vi "Topo & GridSpectr_DriftCorrection_v10.vi"(6 "Internal use":string, 7 "Grid param":T1 {"height (m)" format="%#_6p"; "width (m)" format="%#_6p"; "center Y (m)" format="%#_6p"; "center X (m)" format="%#_6p"}, 8 "Error in (no error)":errorcluster, 9 "Points Y/Index Y":i32, 10 "Points X/Index X":i32, 11 "Method":enum16{"init", "run", "end"}(ring)=enum."end") -> (0 "Error out":errorcluster)   [LabVIEW 2014]
doc: "Example of a measurement VI to be used in the \"Experiments on a Grid\" tool as external VI.\n\nThis example measure the topography and spectroscopy data. The spectroscopy measurements are taken on a subgrid. The data are saved to a sxm and a binary file.\n\n- Nanonis Programming Interface -"
uses:
  <userlib>/Nanonis Prog Interface V5/Scan/Grid/GridPatternGet.vi
  <userlib>/Nanonis Prog Interface V5/Nanonis Prog Interface.lvlib
panel:
  in  "Lockin ON/OFF":bool
  in  "Correct Drift":bool
  in  "Email when finished":string="cornelius.krull@monash.edu"
  in  "STS z offset":dbl=1.15e-09 format="%#_6p"
  out "ETA":timestamp
  out "remaining":dbl format="%<%H:%M:%S>t"
  out "Progress":u8(slide) scale=0.0..100.0 scale format="%#.1g"
  out "total Points":i32
  in  "preSTS delay [ms]":u32=3
  in  "STS Bias":dbl=0.005 format="%#_6p"
  in  "Move Bias":dbl=-0.01 format="%#_6p"
  in  "Move Current":dbl=1.5e-11 format="%#_6p"
  in  "Imaging Bias":dbl=-0.01 format="%#_6p"
  in  "max applied Drift Correction":i32=20 min=1 max=100 step=1 format="%.0p"
  in  "Correlate":u16(ring) items=["first Frame", "successive Frames"]
  out "Topo Images taken":i32=14
  in  "Increment":i32=40
  in  "Threshold":i32=2 min=1 step=1
  in  "tip Speed (m/s)":sgl=1e-08 format="%.2p"
  out "X drift":i32
  out "Y drift":i32
  out "Last Drift detected":i32=40
  in  "MaxImagesBack":i32=40
  in  "Channel index (0-23)":u8=14
  in  "File name":string="single_mol_shortSTS"
  in  "STS Current":dbl=1.15e-09 format="%#_6p"
  in  "Imaging Current":dbl=1.5e-11 format="%#_6p"
  in  "zdrift \nDuration (s)":dbl
  in  "Correct z drift":bool
  out "Status":string="finishing"
  in  "Drift correction Pixels":i32=256 caption="Topo Pixels"
  out "Y Offset":dbl format="%#_6p"
  out "X Offset":dbl format="%#_6p"
  out "Points taken":dbl=14.0
  in  "Drift Correction every":i32=40
  in  "Y subgrid spacing":u16=1
  in  "X subgrid spacing":u16=1
  # "GRID points"
  # "Increase this if no Drift was detected for \na certain number of images"
  # "%"
  # "time (HH:MM:SS)"
  # "images back"
  # "% of image size"
  # "RUN smart tilt before starting the GRID"
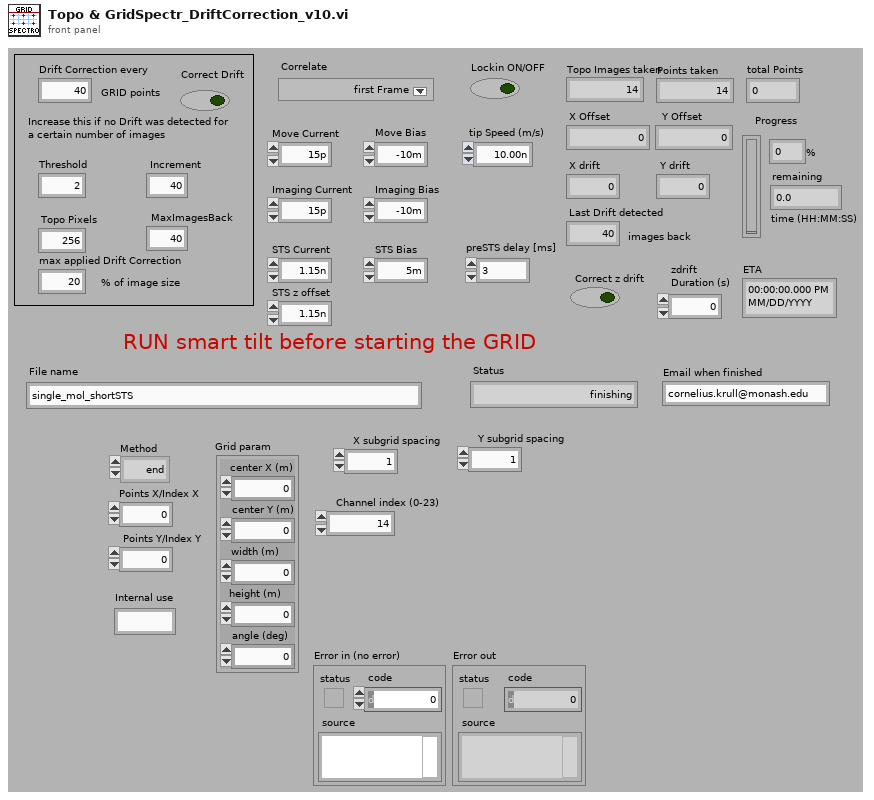
[diagram p1: front panel]
types:
  T1 = cluster{"center X (m)":sgl, "center Y (m)":sgl, "width (m)":sgl, "height (m)":sgl, "angle (deg)":sgl}
  T2 = cluster{"Drift correction Pixels":i32, "Imaging Current":dbl, "STS Current":dbl, "MaxImagesBack":i32, "tip Speed (m/s)":sgl, "Threshold":i32, "Increment":i32, "Correlate":u16, "max applied Drift Correction":i32, "Imaging Bias":dbl, "Move Current":dbl, "Move Bias":dbl, "STS Bias":dbl, "preSTS delay [ms]":u32, "STS z offset":dbl, "Correct Drift":bool, "Lockin ON/OFF":bool}
  T3 = cluster{"center X":sgl, "center Y":sgl, "angle":sgl, "width":sgl, "height":sgl, "# pixels":i32, "# lines":i32}
  T4 = cluster{"Name":string, "Calibration":sgl, "Offset":sgl, "Channel index":i32}[]
  T5 = cluster{"up/down":bool, "time/line":sgl, "start time":timestamp, "end time":timestamp}
  T6 = cluster{"Z averaging time (s)":sgl, "Z offset (m)":sgl, "Initial settling time (s)":sgl}
  T7 = cluster{"Max. slew rate (V/s)":sgl, "Settling time (s)":sgl, "Integration time (s)":sgl}
  T8 = cluster{"End settling time (s)":sgl, "Z control time (s)":sgl}
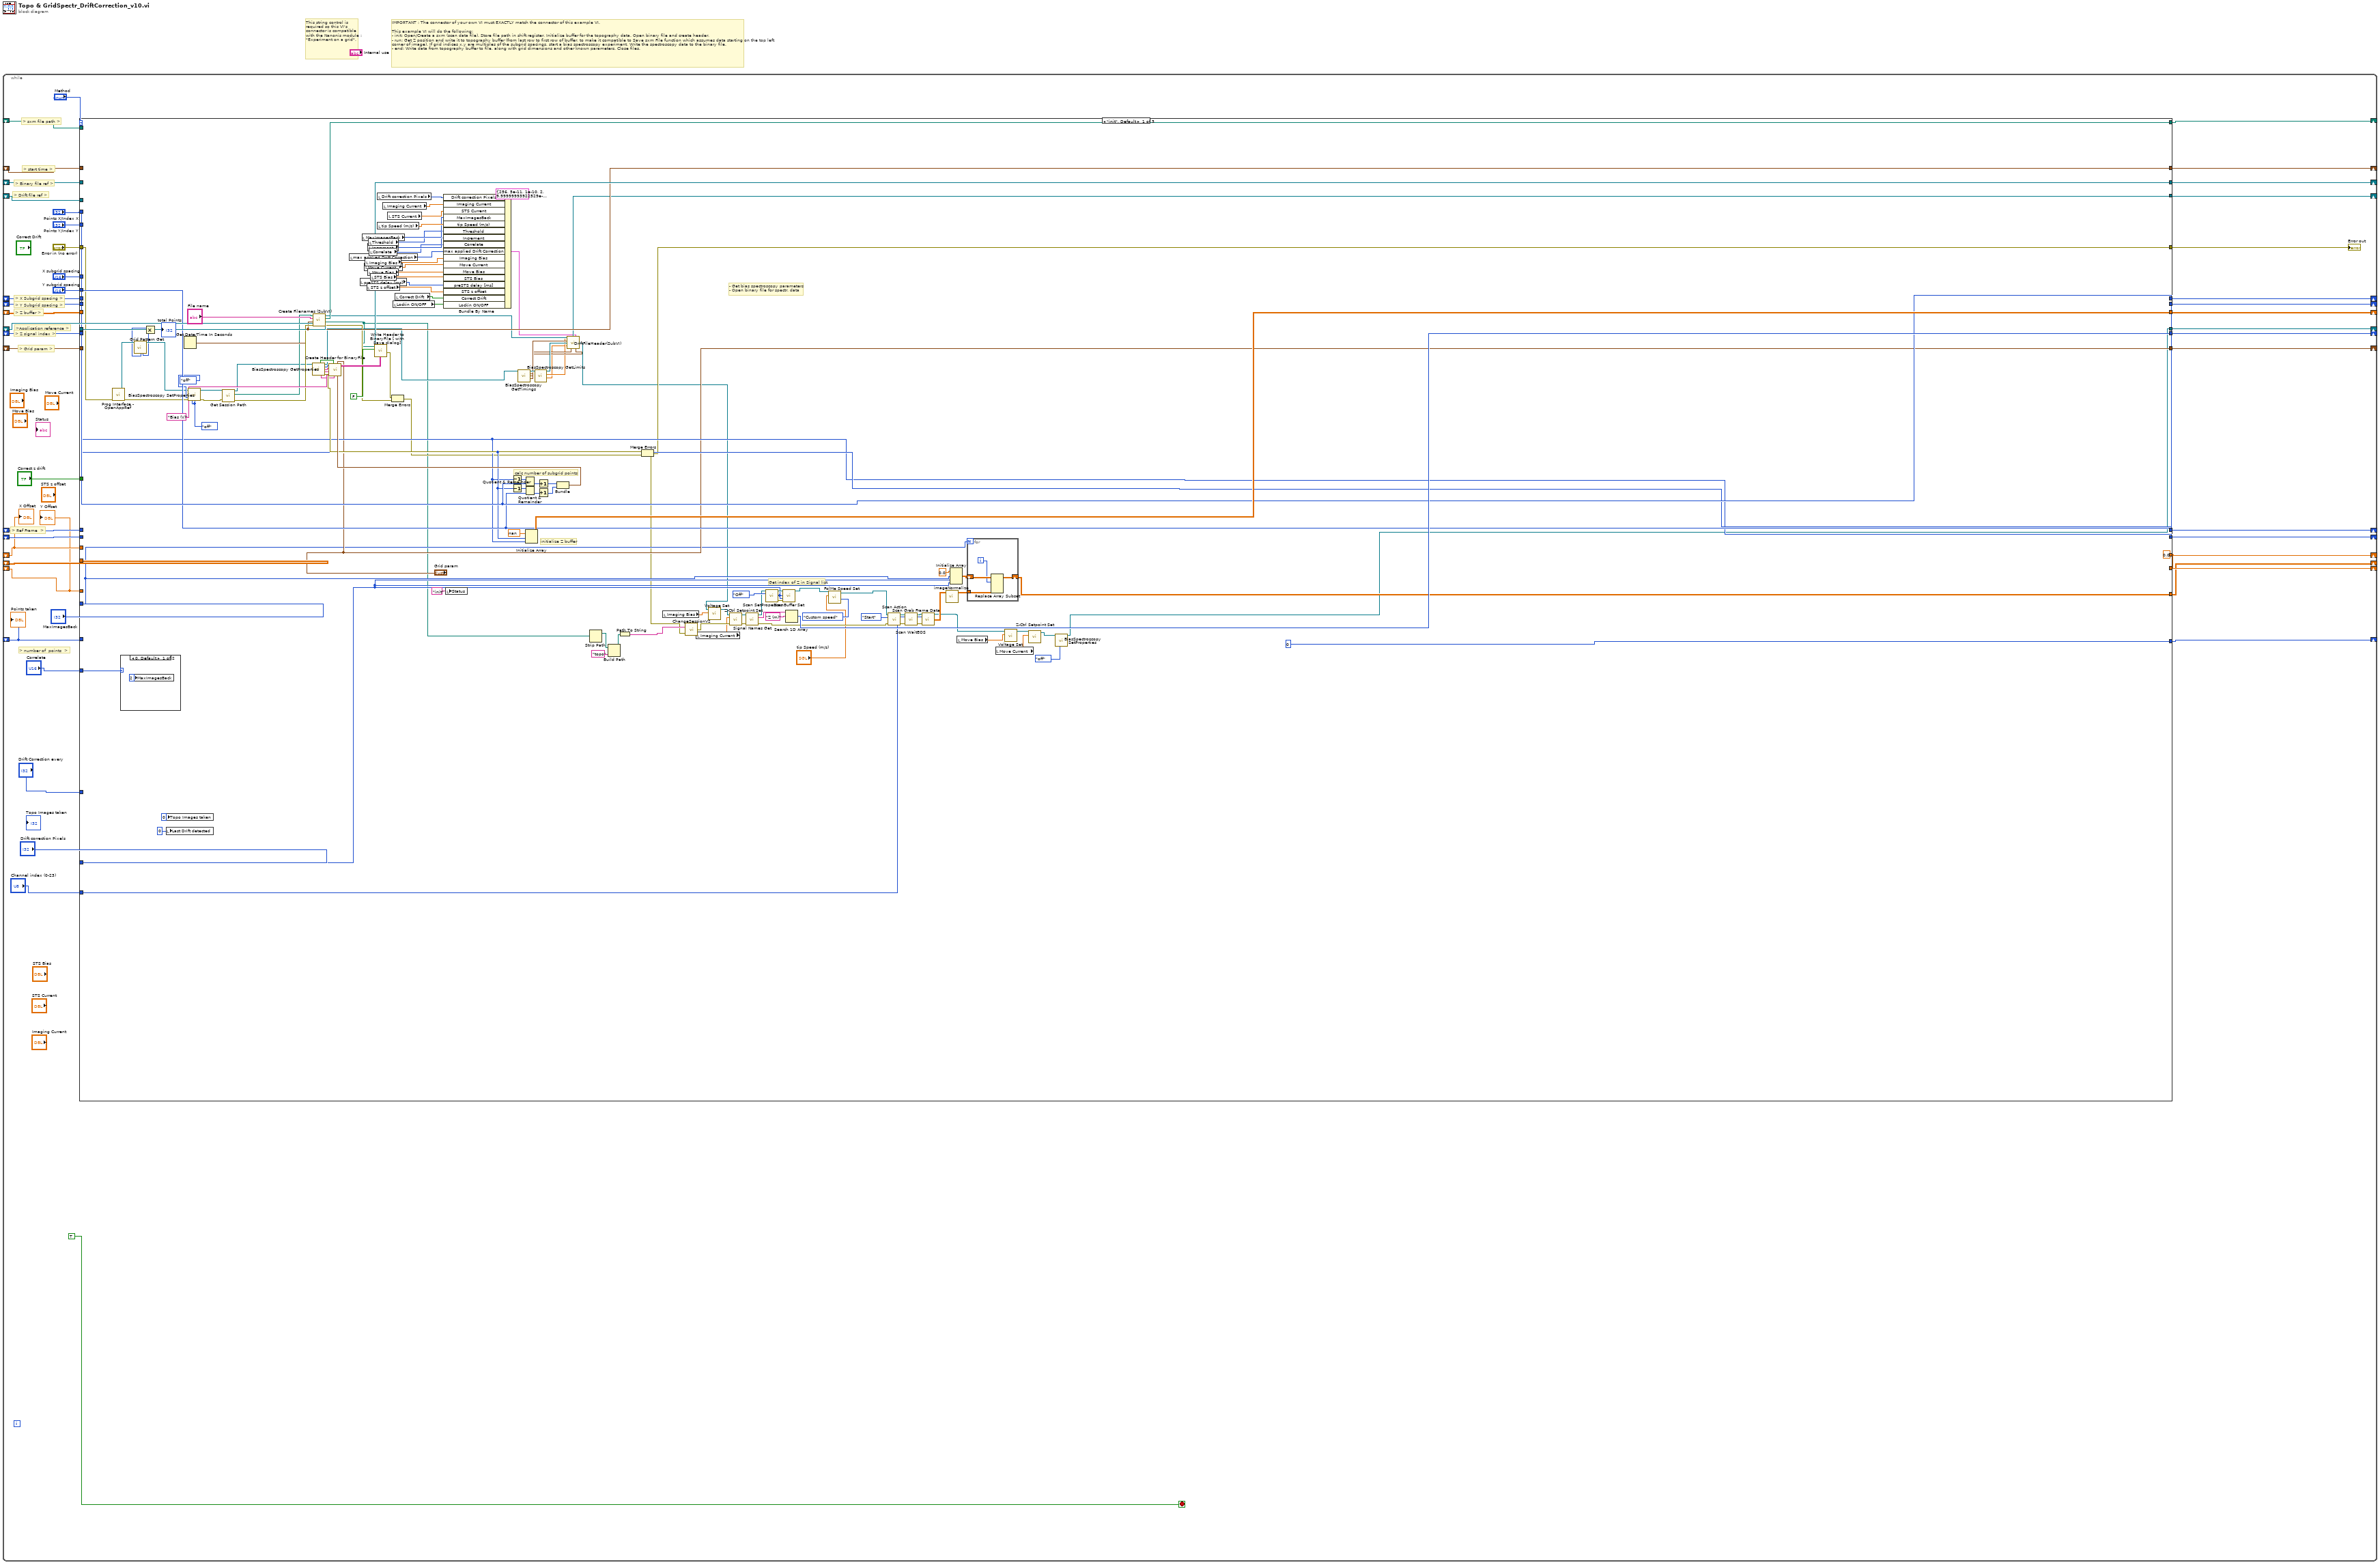
[diagram p0: block diagram]
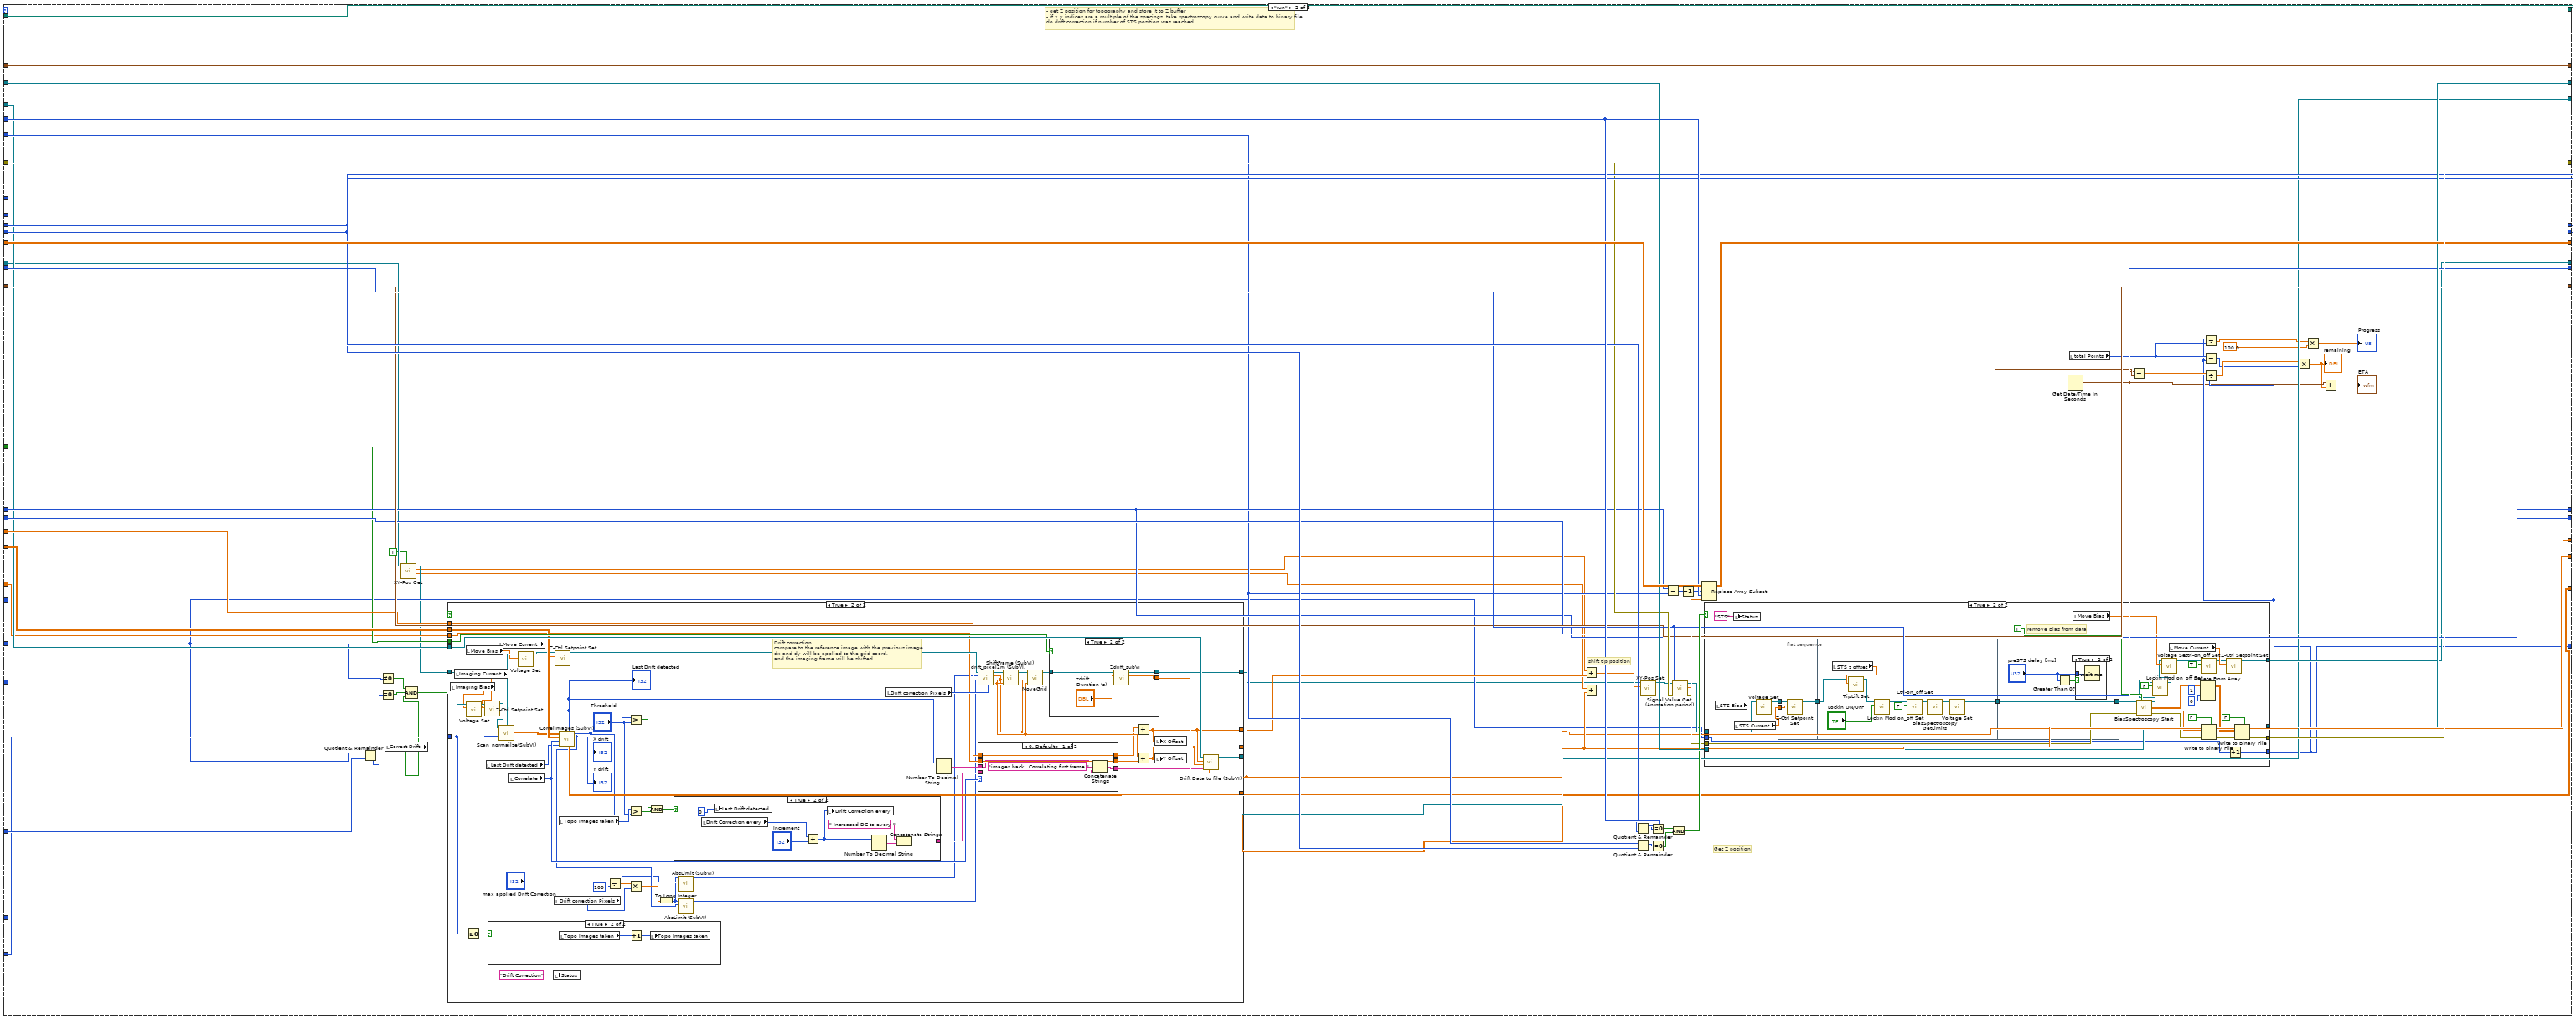
[diagram p3: hidden frame]
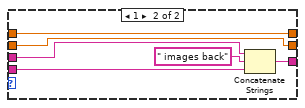
[diagram p5: hidden frame]
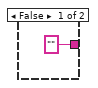
[diagram p7: hidden frame]
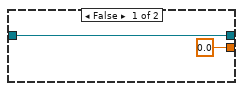
[diagram p8: hidden frame]
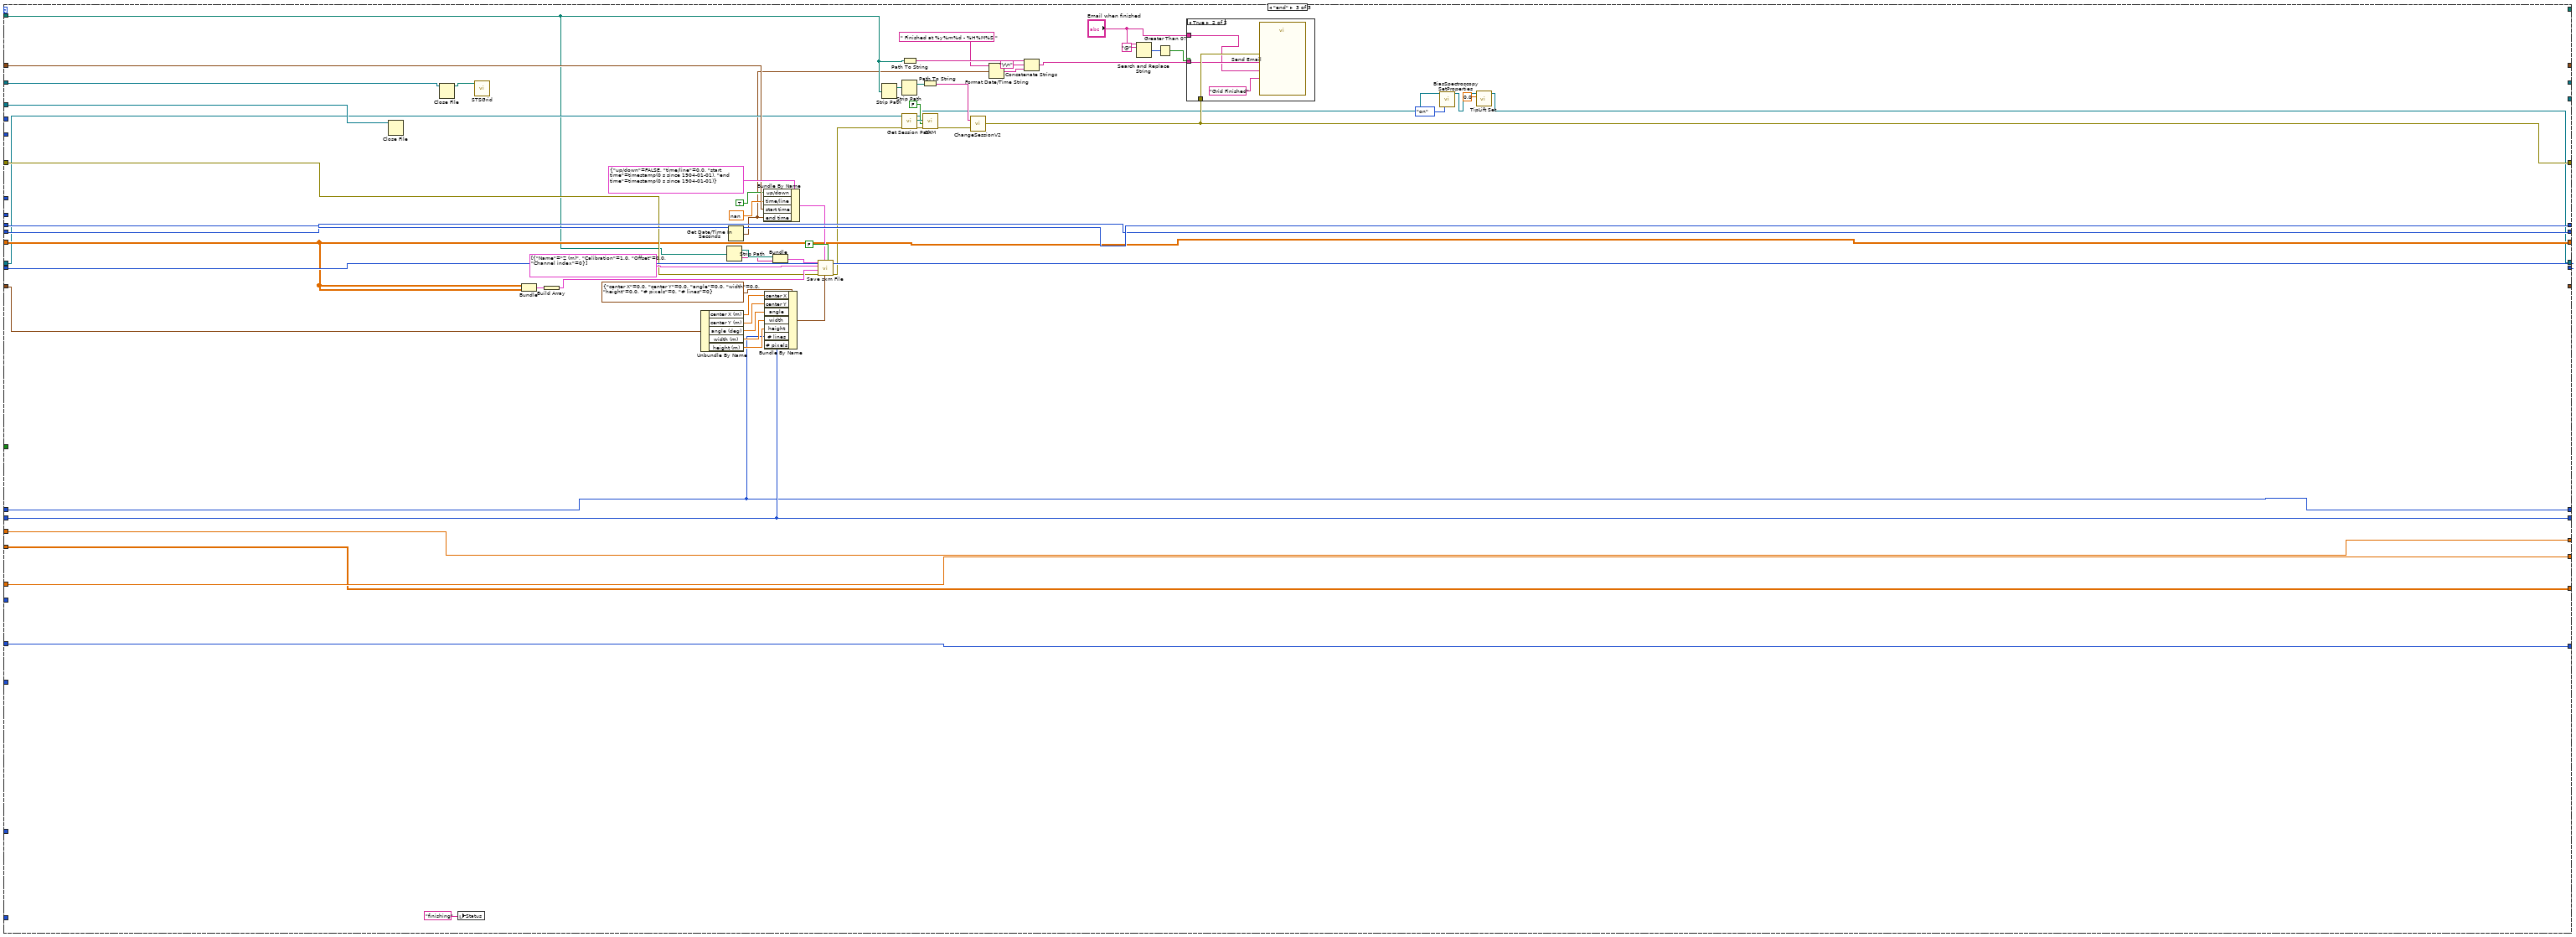
[diagram p11: hidden frame]
diagram:
  # "This string control is required so this VI's connector is compatible with the Nanonis module : \"Experiment on a grid\"."
  # "IMPORTANT : The connector of your own VI must EXACTLY match the connector of this example VI.\n\nThis example VI will do the following:\n- init: Open/Create a sxm (scan data file). Store file path in shift register. Initialize buffer for the topography data. Open binary file and create header.\n- run: Get Z position and write it to topography buffer (from last row to first row of buffer, to make it compatible to Save sxm File function which assumes data starting on the top left corner of image). If grid indices x,y are multiples of the subgrid spacings, start a bias spectroscopy experiment. Write the spectroscopy data to the binary file.\n- end: Write data from topography buffer to file, along with grid dimensions and other known parameters. Close files."
  n1 = while {
    shift-right: [w21] -> _
    shift-left: _ -> [w44]
    shift-right: [w39] -> _
    shift-left: _ -> [w38]
    shift-right: [w36] -> _
    shift-left: _ -> [w37]
    shift-right: [w35] -> _
    shift-left: _ -> [w34]
    shift-right: [w28] -> _
    shift-left: _ -> [w30]
    shift-right: [w29] -> _
    shift-left: _ -> [w31]
    shift-right: [w27] -> _
    shift-left: _ -> [w26]
    shift-right: [w25] -> _
    shift-left: _ -> [w24]
    shift-right: [w23] -> _
    shift-left: _ -> [w22]
    shift-right: [w20] -> _
    shift-left: _ -> [w19]
    shift-right: [w18] -> _
    shift-left: _ -> [w17]
    shift-right: [w16] -> _
    shift-left: _ -> [w9]
    shift-right: [w15] -> _
    shift-left: _ -> [w8]
    shift-right: [w14] -> _
    shift-left: _ -> [w11]
    shift-right: [w13] -> _
    shift-left: _ -> [w10]
    shift-right: [w6] -> _
    shift-left: _ -> [w5]
    stop <- TRUE stop-if-true
    # "> Drift file ref >"
    # "> number of  points  >"
    # "> Ref Frame  >"
    # "> Grid param >"
    # "> start time >"
    # ">Application reference >"
    # "> Y Subgrid spacing >"
    # "> X Subgrid spacing >"
    # "> Z signal index >"
    # "> Binary file ref >"
    # "> Z buffer >"
    # "> sxm file path >"
    n2 = case shown="\"init\", Default" "Method" {
      tunnel: [w125 w239 _] -> w21
      tunnel: w44 -> [_ w239 w397]
      tunnel: "Error in (no error)" -> [w127 w225 w428]
      tunnel: [w101 w238 w398] -> w42
      tunnel: "Points X/Index X" -> [w146 w233 _]
      tunnel: "Points Y/Index Y" -> [w147 w218 _]
      tunnel: [w170 w236 w417] -> w39
      tunnel: w38 -> [_ w237 w417]
      tunnel: w37 -> [_ w235 w410]
      tunnel: [w162 w234 _] -> w36
      tunnel: [w160 w223 w442] -> w35
      tunnel: w34 -> [_ w223 w442]
      tunnel: "X subgrid spacing" -> [w159 _ _]
      tunnel: "Y subgrid spacing" -> [w158 _ _]
      tunnel: w31 -> [_ w227 w441]
      tunnel: w30 -> [_ w226 w440]
      tunnel: [w159 w227 w441] -> w29
      tunnel: [w158 w226 w440] -> w28
      tunnel: [w78 w211 w383] -> w27
      tunnel: w26 -> [_ w194 w403]
      tunnel: ["Grid param" w221 _] -> w25
      tunnel: w24 -> [_ w221 w427]
      tunnel: [w124 w184 _] -> w23
      tunnel: w22 -> [_ w184 w435]
      tunnel: [w147 w219 w418] -> w20
      tunnel: w19 -> [_ w219 w418]
      tunnel: [w146 w220 w419] -> w18
      tunnel: w17 -> [_ w220 w419]
      tunnel: [w137 w201 w416] -> w16
      tunnel: [w137 w206 w414] -> w15
      tunnel: [w119 w200 w411] -> w14
      tunnel: [0 w182 w415] -> w13
      tunnel: w10 -> [_ w197 w415]
      tunnel: "Drift Correction every" -> [_ w214 _]
      tunnel: w11 -> [_ w205 w411]
      tunnel: w9 -> [_ w212 w416]
      tunnel: w8 -> [_ w198 w414]
      tunnel: "Drift correction Pixels" -> [w118 _ _]
      tunnel: [w73 w203 _] -> w6
      tunnel: w5 -> [_ w204 w412]
      tunnel: "Correct z drift" -> [_ w202 _]
      tunnel: "Channel index (0-23)" -> [w122 w199 _]
      tunnel: "MaxImagesBack" -> [w117 _ _]
      tunnel: "Correlate" -> [w93 _ _]
      frame "init", Default {
        w75 = enum16{"no change", "on", "off"}."off" ("Save dialog")
        w137 = 0.0
        # "- Get bias spectroscopy parameters\n- Open binary file for spectr. data"
        # "initialize Z buffer"
        # "calc number of subgrid points"
        # "Get index of Z in Signal list"
        n3 = call <userlib>:"Prog Interface - OpenAppRef.vi"("Error in (no error)"=w127) -> ("Error out"=w99:errorcluster, "Application reference"=w83:refnum<vi>)  [unwired: 5 in]
        n4 = case shown="0, Default" w93 {
          frame 0, Default {
            n5 = local write "MaxImagesBack"(2 ("StepsBack")) -> ()
          }
          frame 1 {
          }
        }
        n6 = call-poly <userlib>:"Grid Pattern Get.vi"("Application ref in"=w83) -> ("Points Y"=w80:i32, "Points X"=w81:i32, "Application ref out"=w82:refnum<vi>)  [unwired: 10 in, 6 out]
        n7 = Multiply(x=w80, y=w81) -> (x*y=→"total Points":i32)
        n8 = local write "Topo Images taken"(0 ("Images taken")) -> ()
        n9 = local write "Last Drift detected"(0 ("Last Drift detected")) -> ()
        n10 = Get Date/Time In Seconds() -> (seconds since 1Jan1904=w124:timestamp)
        n11 = call <userlib>:"BiasSpectroscopy SetProperties.vi"("Application ref in"=w82, "Autosave (no change)"=enum16{"no change", "on", "off"}."off", "Error in (no error)"=w99, "Z-Controller hold (no change)"=w75, "Save dialog"=w75) -> ("Application ref out"=w96:refnum<vi>, "Error out"=w95:errorcluster)  [unwired: 9 in]
        n12 = call <userlib>:"Get Session Path.vi"("error in (no error)"=w95, "Application ref in"=w96) -> ("error out"=w126:errorcluster, "Session path"=w107:path, "Application ref out"=w97:refnum<vi>)  [unwired: 7 in]
        n13 = call <userlib>:"BiasSpectroscopy GetProperties.vi"("Application ref in"=w97) -> ("Backward sweep"=w166:bool, "Application ref out"=w111:refnum<vi>, "Number of points"=w149:i32, "Channels"=w148:string[], "Parameters"=w164:string[], "Fixed parameters"=w151:string[], "Error out"=w163:errorcluster)  [unwired: 6 in, 2 out]
        n14 = call "Create Filenames (SubVI).vi"("error in (no error)"=w126, "seconds since 1Jan1904"=w124, "File name"="File name", "Session path"=w107) -> ("error out"=w112:errorcluster, "binFilePath"=w103:path, "topoFilePath"=w125:path, "Drift File out"=w74:refnum<file>)  [unwired: 4 in]
        n15 = local read "max applied Drift Correction"() -> (w54:i32)
        n16 = local read "preSTS delay [ms]"() -> (w49:u32)
        n17 = local read "MaxImagesBack"() -> (w58:i32)
        n18 = local read "Move Current"() -> (w52:dbl)
        n19 = local read "Imaging Bias"() -> (w53:dbl)
        n20 = local read "STS z offset"() -> (w48:dbl)
        n21 = local read "Increment"() -> (w56:i32)
        n22 = local read "Move Bias"() -> (w51:dbl)
        n23 = local read "Threshold"() -> (w57:i32)
        n24 = local read "Correlate"() -> (w55:u16)
        n25 = local read "STS Bias"() -> (w50:dbl)
        n26 = local read "Drift correction Pixels"() -> (w63:i32)
        n27 = local read "tip Speed (m/s)"() -> (w60:sgl)
        n28 = local read "Imaging Current"() -> (w62:dbl)
        n29 = local read "STS Current"() -> (w61:dbl)
        n30 = local read "Lockin ON/OFF"() -> (w59:bool)
        n31 = local read "Correct Drift"() -> (w47:bool)
        n32 = Bundle By Name(cluster=T2 {"Drift correction Pixels"=256, "Imaging Current"=5e-11, "STS Current"=1e-10, "MaxImagesBack"=2, "tip Speed (m/s)"=1e-08, "Threshold"=2, "Increment"=64, "Correlate"=0, "max applied Drift Correction"=20, "Imaging Bias"=-0.02, "Move Current"=1.5e-11, "Move Bias"=-0.02, "STS Bias"=0.1, "preSTS delay [ms]"=1000, "STS z offset"=-1.7e-10, "Correct Drift"=TRUE, "Lockin ON/OFF"=TRUE} ("Drift Correction"), "Drift correction Pixels"=w63, "Imaging Current"=w62, "STS Current"=w61, "MaxImagesBack"=w58, "tip Speed (m/s)"=w60, "Threshold"=w57, "Increment"=w56, "Correlate"=w55, "max applied Drift Correction"=w54, "Imaging Bias"=w53, "Move Current"=w52, "Move Bias"=w51, "STS Bias"=w50, "preSTS delay [ms]"=w49, "STS z offset"=w48, "Correct Drift"=w47, "Lockin ON/OFF"=w59) -> (w65:T2)
        n33 = local write "Status"("init" ("Status")) -> ()
        n34 = Decrement(x=w146) -> (x-1=w157:i32)
        n35 = Decrement(x=w147) -> (x-1=w156:i32)
        n36 = call <userlib>:"BiasSpectroscopy GetTimings.vi"("Application ref in"=w111) -> ("Application ref out"=w115:refnum<vi>, "Initialization"=w68:T6, "Sweep Timing"=w69:T7, "End of Sweep"=w70:T8)  [unwired: 10 in, 1 out]
        n37 = Quotient & Remainder(x=w157, y=w159) -> (floor(x/y)=w155:i32)  [unwired: 1 out]
        n38 = Quotient & Remainder(x=w156, y=w158) -> (floor(x/y)=w154:i32)  [unwired: 1 out]
        n39 = Initialize Array(sgl nan ("element"), w147, w146) -> (w170:sgl[][])
        n40 = call <userlib>:"BiasSpectroscopy GetLimits.vi"("Application ref in"=w115) -> ("End value (V)"=w66:sgl, "Start value (V)"=w67:sgl, "Application ref out"=w72:refnum<vi>)  [unwired: 5 in, 1 out]
        n41 = Increment(x=w155) -> (x+1=w153:i32)
        n42 = Increment(x=w154) -> (x+1=w152:i32)
        n43 = Bundle(w153, w152) -> (w165:cluster{i32, i32})  [unwired: 1 in]
        n44 = call <userlib>:"Create Header for BinaryFile.vi"("Grid points"=w165, "Grid param"="Grid param", "Fixed parameters"=w151, "Backward sweep"=w166, "Sweep signal"="Bias (V)" ("Sweep Signal"), "Parameters"=w164, "Channels"=w148, "Points per sweep"=w149) -> ("Header (fixed attributes)"=w168:string[][])  [unwired: 3 in]
        n45 = call <userlib>:"Write Header to BinaryFile [ with Save dialog].vi"("Fixed Attributes"=w168, "Show Dialog? (T)"=FALSE, "Filename"=w103) -> ("Error out"=w113:errorcluster, "File ref"=w162:refnum<file>)  [unwired: 5 in, 2 out]
        n46 = Merge Errors(w113, w112) -> (w114:errorcluster)
        n47 = call "DriftFileHeader(SubVI).vi"("Start value (V)"=w67, "Byte Stream File in"=w74, "Drift Correction"=w65, "End of Sweep"=w70, "Application ref in"=w72, "End value (V)"=w66, "Sweep Timing"=w69, "Initialization"=w68) -> ("Byte Stream File out"=w73:refnum<file>, "Application ref out"=w71:refnum<vi>)  [unwired: 6 in]
        n48 = Strip Path(path=w103) -> (stripped path=w106:path)  [unwired: 1 out]
        n49 = Build Path(base path=w106, name or relative path="topo") -> (appended path=w104:path)
        n50 = Path To String(path=w104) -> (string=w102:string)
        n51 = Merge Errors(w163, w114) -> (w101:errorcluster)
        n52 = local read "Imaging Bias"() -> (w86:dbl)
        n53 = call "ChangeSessionV2.vi"("error in (no error)"=w101, "Session"=w102) -> ("error out"=w100:errorcluster)
        n54 = local read "Imaging Current"() -> (w85:dbl)
        n55 = call <userlib>:"Voltage Set.vi"("Bias (V)"=w86, "Application ref in"=w71) -> ("Application ref out"=w89:refnum<vi>)  [unwired: 8 in, 1 out]
        n56 = call <userlib>:"Z-Ctrl Setpoint Set.vi"("error in (no error)"=w100, "Z Controller setpoint"=w85, "Application ref in"=w89) -> ("error out"=w128:errorcluster, "Application ref out"=w129:refnum<vi>)  [unwired: 7 in]
        n57 = call <userlib>:"Signal Names Get.vi"("error in (no error)"=w128, "Application ref in"=w129) -> ("error out"=w138:errorcluster, "Signals Names"=w150:string[], "Application ref out"=w133:refnum<vi>)  [unwired: 5 in]
        n58 = call <userlib>:"Scan SetProperties.vi"("Application ref in"=w133, "Continuous scan"=enum16{"No change", "On", "Off"}."Off") -> ("Application ref out"=w135:refnum<vi>, "Error out"=w134:errorcluster)  [unwired: 12 in]
        n59 = call <userlib>:"ScanBuffer Set.vi"("Application ref in"=w135, "Pixels"=w118, "Lines"=w118, "error in (no error)"=w134) -> ("Application ref out"=w91:refnum<vi>)  [unwired: 10 in, 1 out]
        n60 = Search 1D Array(1D array=w150, element="Z (m)") -> (index of element=w160:i32)  [unwired: 1 in]
        n61 = call <userlib>:"FolMe Speed Set.vi"("Speed Setting (Custom)"=enum32{"Scan speed", "Custom speed"}."Custom speed", "Speed (m/s)"="tip Speed (m/s)", "Application ref in"=w91) -> ("Application ref out"=w110:refnum<vi>)  [unwired: 5 in, 1 out]
        n62 = call <userlib>:"Scan Action.vi"("error in (no error)"=w138, "Scan action (Start)"=enum16{"Start", "Stop", "Pause", "Resume"}."Start", "Application ref in"=w110) -> ("error out"=w144:errorcluster, "Application ref out"=w143:refnum<vi>)  [unwired: 6 in]
        n63 = call <userlib>:"Scan WaitEOS.vi"("error in (no error)"=w144, "Application ref in"=w143) -> ("error out"=w141:errorcluster, "Application ref out"=w142:refnum<vi>)  [unwired: 5 in, 2 out]
        n64 = call <userlib>:"Scan Grab Frame Data.vi"("Application ref in"=w142, "Channel index (0-23)"=w122, "error in (no error)"=w141) -> ("Application ref out"=w84:refnum<vi>, "Scan frame data"=w130:sgl[][])  [unwired: 8 in, 3 out]
        n65 = call "imageNormalize.vi"("Data"=w130) -> ("Array"=w116:dbl[][])  [unwired: 10 in]
        n66 = Initialize Array(0.0 ("element"), w117, w118, w118) -> (w120:dbl[][][])
        n67 = local read "Move Bias"() -> (w88:dbl)
        n68 = for {
          N: w117 -> [_]
          tunnel: w116 -> [w174]
          shift-right: [w173] -> w119
          shift-left: w120 -> [w175]
          i -> [w172]
          n69 = Replace Array Subset(array=w175, new element=w174, index (dim 0)=w172) -> (w173:dbl[][][])  [unwired: 2 in]
        }
        n70 = local read "Move Current"() -> (w87:dbl)
        n71 = call <userlib>:"Voltage Set.vi"("Bias (V)"=w88, "Application ref in"=w84) -> ("Application ref out"=w90:refnum<vi>)  [unwired: 8 in, 1 out]
        n72 = call <userlib>:"Z-Ctrl Setpoint Set.vi"("Z Controller setpoint"=w87, "Application ref in"=w90) -> ("Application ref out"=w77:refnum<vi>)  [unwired: 8 in, 1 out]
        n73 = call <userlib>:"BiasSpectroscopy SetProperties.vi"("Application ref in"=w77, "Z-Controller hold (no change)"=enum16{"no change", "on", "off"}."off") -> ("Application ref out"=w78:refnum<vi>)  [unwired: 12 in, 1 out]
      }
      frame "run" {
        # "shift tip position"
        # "Get Z position"
        # "- get Z position for topography and store it to Z buffer\n- if x,y indices are a multiple of the spacings, take spectroscopy curve and write data to binary file\ndo drift correction if number of STS position was reached"
        n74 = Quotient & Remainder(x=w197, y=w214) -> (x-y*floor(x/y)=w215:i32)  [unwired: 1 out]
        n75 = Not Equal To 0?(x=w197) -> (x != 0?=w195:bool)
        n76 = Equal To 0?(x=w215) -> (x = 0?=w213:bool)
        n77 = local read "Correct Drift"() -> (w176:bool)
        n78 = call <userlib>:"XY-Pos Get.vi"("Wait for newest data (F=False)"=TRUE, "Application ref in"=w194) -> ("Y (m)"=w190:sgl, "X (m)"=w191:sgl, "Application ref out"=w193:refnum<vi>)  [unwired: 5 in, 1 out]
        n79 = Compound Arithmetic op=AND(w195, w213, w176) -> (w196:bool)
        n80 = case shown="True" w196 {
          tunnel: w193 -> [w244 w252]
          tunnel: [w244 w294] -> w189
          tunnel: w205 -> [w241 w289]
          tunnel: [w243 w292] -> w201
          tunnel: [w242 w291] -> w206
          tunnel: w212 -> [w243 w268]
          tunnel: w198 -> [w242 w266]
          tunnel: [w241 w285] -> w200
          tunnel: w204 -> [w240 w297]
          tunnel: [w240 w296] -> w203
          tunnel: w202 -> [_ w293]
          tunnel: w199 -> [_ w272]
          frame False {
          }
          frame True {
            # "Drift correction \ncompare to the reference image with the previous image \ndx and dy will be applied to the grid coord, \nand the imaging frame will be shifted"
            n81 = local read "Imaging Bias"() -> (w250:dbl)
            n82 = local read "Imaging Current"() -> (w249:dbl)
            n83 = local read "Move Bias"() -> (w246:dbl)
            n84 = Greater Or Equal To 0?(x=w272) -> (x >= 0?=w271:bool)
            n85 = call <userlib>:"Voltage Set.vi"("Bias (V)"=w250, "Application ref in"=w252) -> ("Application ref out"=w251:refnum<vi>)  [unwired: 8 in, 1 out]
            n86 = call <userlib>:"Z-Ctrl Setpoint Set.vi"("Z Controller setpoint"=w249, "Application ref in"=w251) -> ("Application ref out"=w290:refnum<vi>)  [unwired: 8 in, 1 out]
            n87 = local read "Last Drift detected"() -> (w263:i32)
            n88 = case shown="True" w271 {
              frame False {
              }
              frame True {
                n89 = local read "Topo Images taken"() -> (w312:i32)
                n90 = Increment(x=w312) -> (x+1=w311:i32)
                n91 = local write "Topo Images taken"(w311) -> ()
              }
            }
            n92 = local read "Move Current"() -> (w245:dbl)
            n93 = call "Scan_normailze(SubVI).vi"("Channel index (0-23)"=w272, "Application in"=w290) -> ("Array"=w286:dbl[][], "Application out"=w247:refnum<vi>)  [unwired: 7 in, 1 out]
            n94 = local read "Correlate"() -> (w269:u16)
            n95 = call <userlib>:"Voltage Set.vi"("Bias (V)"=w246, "Application ref in"=w247) -> ("Application ref out"=w248:refnum<vi>)  [unwired: 8 in, 1 out]
            n96 = local write "Status"("Drift Correction" ("Status")) -> ()
            n97 = local read "Drift correction Pixels"() -> (w260:i32)
            n98 = call <userlib>:"Z-Ctrl Setpoint Set.vi"("Z Controller setpoint"=w245, "Application ref in"=w248) -> ("Application ref out"=w281:refnum<vi>)  [unwired: 8 in, 1 out]
            n99 = local read "Topo Images taken"() -> (w274:i32)
            n100 = call "CorrelImages (SubVI).vi"("last drift detected"=w263, "Correlate"=w269, "Ref Array"=w289, "New Image"=w286) -> ("Y drift"=w257:i32, "X drift"=w254:i32, "Ref Array out"=w285:dbl[][][], "Queue Steps"=w270:i32)  [unwired: 4 in]
            "X drift" <- w254
            "Y drift" <- w257
            "Last Drift detected" <- w270
            n101 = Divide(x="max applied Drift Correction", y=100) -> (x/y=w259:dbl)
            n102 = Greater Or Equal?(x=w270, y="Threshold") -> (x >= y?=w276:bool)
            n103 = Greater?(x=w274, y="Threshold") -> (0:w273:bool)
            n104 = Multiply(x=w259, y=w260) -> (x*y=w261:dbl)
            n105 = And(x=w276, y=w273) -> (x .and. y?=w275:bool)
            n106 = To Long Integer(number=w261) -> (32bit integer=w253:i32)
            n107 = case shown="True" w275 {
              tunnel: ["" w316] -> w277
              frame False {
              }
              frame True {
                n108 = local read "Drift Correction every"() -> (w315:i32)
                n109 = local write "Last Drift detected"(0 ("Last Drift detected")) -> ()
                n110 = Add(x=w315, y="Increment") -> (x+y=w319:i32)
                n111 = local write "Drift Correction every"(w319) -> ()
                n112 = Number To Decimal String(number=w319) -> (decimal integer string=w318:string)  [unwired: 1 in]
                n113 = Concatenate Strings(" Increased DC to every " ("string"), w318) -> (w316:string)
              }
            }
            n114 = call "AbsLimit (SubVI).vi"("in"=w254, "Abslimt"=w253) -> ("Numeric out"=w256:i32)  [unwired: 9 in]
            n115 = call "AbsLimit (SubVI).vi"("in"=w257, "Abslimt"=w253) -> ("Numeric out"=w255:i32)  [unwired: 9 in]
            n116 = local read "Drift correction Pixels"() -> (w282:i32)
            n117 = Number To Decimal String(number=w270) -> (decimal integer string=w288:string)  [unwired: 1 in]
            n118 = call "drift_pixel2m (SubVI).vi"("Application in"=w281, "X drift"=w256, "Y drift"=w255, "Drift correction Pixels"=w282) -> ("Application out"=w280:refnum<vi>, "x drift"=w278:sgl, "y drift"=w279:sgl)  [unwired: 2 in, 1 out]
            n119 = case shown="0, Default" w269 {
              tunnel: w288 -> [w299 w310]
              tunnel: [w304 w309] -> w287
              tunnel: w277 -> [w302 w307]
              tunnel: w268 -> [w300 w306]
              tunnel: [w300 w306] -> w267
              tunnel: w266 -> [w301 w305]
              tunnel: [w301 w305] -> w265
              frame 0, Default {
                n120 = Concatenate Strings(w299, "images back , Correlating first frame " ("string"), w302) -> (w304:string)
              }
              frame 1 {
                n121 = Concatenate Strings(w310, " images back" ("string"), w307) -> (w309:string)
              }
            }
            n122 = call "ShiftFrame (SubVI).vi"("Y shift"=w279, "X shift"=w278, "Application in"=w280) -> ("Application out"=w284:refnum<vi>)  [unwired: 8 in]
            n123 = call "MoveGrid.vi"("y"=w279, "x"=w278, "Application ref in"=w284) -> ("Application ref out"=w283:refnum<vi>)  [unwired: 7 in, 1 out]
            n124 = case shown="True" w293 {
              tunnel: [0.0 ("z drift") w326] -> w295
              tunnel: w283 -> [w321 w325]
              tunnel: [w321 w324] -> w294
              frame False {
              }
              frame True {
                n125 = call "Zdrift_subVi.vi"("Duration"="zdrift \nDuration (s)", "Application in"=w325) -> ("z drift"=w326:dbl, "Application out"=w324:refnum<vi>)  [unwired: 7 in, 1 out]
              }
            }
            n126 = Add(x=w267, y=w278) -> (x+y=w292:dbl)
            n127 = Add(x=w279, y=w265) -> (x+y=w291:dbl)
            n128 = local write "X Offset"(w292) -> ()
            n129 = local write "Y Offset"(w291) -> ()
            n130 = call "Drift Data to file (SubVI).vi"("z drift"=w295, "Comment"=w287, "y Drift"=w291, "X drift"=w292, "Byte Stream File in"=w297) -> ("Byte Stream File out"=w296:refnum<file>)  [unwired: 6 in]
          }
        }
        n131 = Add(x=w191, y=w201) -> (x+y=w208:dbl)
        n132 = Add(x=w190, y=w206) -> (x+y=w207:dbl)
        n133 = Quotient & Remainder(x=w233, y=w227) -> (x-y*floor(x/y)=w232:i32)  [unwired: 1 out]
        n134 = Quotient & Remainder(x=w218, y=w226) -> (x-y*floor(x/y)=w231:i32)  [unwired: 1 out]
        n135 = call <userlib>:"XY-Pos Set.vi"("Y (m)"=w207, "X (m)"=w208, "Application ref in"=w189) -> ("Application ref out"=w209:refnum<vi>)  [unwired: 5 in, 1 out]
        n136 = Equal To 0?(x=w232) -> (x = 0?=w230:bool)
        n137 = Equal To 0?(x=w231) -> (x = 0?=w229:bool)
        n138 = Subtract(x=w219, y=w218) -> (x-y=w217:i32)
        n139 = And(x=w230, y=w229) -> (x .and. y?=w228:bool)
        n140 = call <userlib>:"Signal Value Get (Animation period).vi"("error in (no error)"=w225, "Signal index (0-47)"=w223, "Application ref in"=w209) -> ("error out"=w224:errorcluster, "Signal value"=w222:sgl, "Application ref out"=w210:refnum<vi>)  [unwired: 5 in]
        n141 = Decrement(x=w217) -> (x-1=w216:i32)
        n142 = Replace Array Subset(array=w237, new element=w222, index (row)=w216, index (col)=w233) -> (w236:sgl[][])
        n143 = case shown="True" w228 {
          tunnel: [w329 w350] -> w238
          tunnel: w235 -> [w330 w364]
          tunnel: [w330 w362] -> w234
          tunnel: w224 -> [w329 w361]
          tunnel: w210 -> [w328 w346]
          tunnel: [w328 w341] -> w211
          tunnel: [w327 w348] -> w182
          tunnel: w197 -> [w327 w349]
          frame False {
            # "Point indices aren't multiple of subgrid spacing\n=> no spectroscopy at this point"
          }
          frame True {
            # "remove Bias from data"
            n144 = local read "STS Bias"() -> (w343:dbl)
            n145 = local write "Status"("STS" ("Status")) -> ()
            n146 = local read "STS Current"() -> (w342:dbl)
            n147 = call <userlib>:"Voltage Set.vi"("Bias (V)"=w343, "Application ref in"=w346) -> ("Application ref out"=w345:refnum<vi>)  [unwired: 8 in, 1 out]
            n148 = flat-sequence {
              tunnel: w345 -> [w367]
              tunnel: w342 -> [w365]
              tunnel: [w366] -> w338
              tunnel: w338 -> [w370]
              tunnel: [w368] -> w337
              tunnel: [w380] -> w344
              tunnel: w337 -> [w380]
              frame #0 {
                n149 = call <userlib>:"Z-Ctrl Setpoint Set.vi"("Z Controller setpoint"=w365, "Application ref in"=w367) -> ("Application ref out"=w366:refnum<vi>)  [unwired: 8 in, 1 out]
              }
              frame #1 {
                n150 = local read "STS z offset"() -> (w373:dbl)
                n151 = call <userlib>:"TipLift Set.vi"("TipLift (m)"=w373, "Application ref in"=w370) -> ("Application ref out"=w369:refnum<vi>)  [unwired: 8 in, 1 out]
                n152 = call <userlib>:"Lockin Mod on_off Set.vi"("Lockin ON/OFF"="Lockin ON/OFF", "Application ref in"=w369) -> ("Application ref out"=w372:refnum<vi>)  [unwired: 8 in, 1 out]
                n153 = call <userlib>:"Ctrl-on_off Set.vi"("Z Controller ON/OFF"=FALSE, "Application ref in"=w372) -> ("Application ref out"=w375:refnum<vi>)  [unwired: 8 in, 1 out]
                n154 = call <userlib>:"BiasSpectroscopy GetLimits.vi"("Application ref in"=w375) -> ("Start value (V)"=w374:sgl, "Application ref out"=w376:refnum<vi>)  [unwired: 5 in, 2 out]
                n155 = call <userlib>:"Voltage Set.vi"("Bias (V)"=w374, "Application ref in"=w376) -> ("Application ref out"=w368:refnum<vi>)  [unwired: 8 in, 1 out]
              }
              frame #2 {
                n156 = Greater Than 0?(x="preSTS delay [ms]") -> (x > 0?=w378:bool)
                n157 = case shown="True" w378 {
                  tunnel: "preSTS delay [ms]" -> [_ w381]
                  frame False {
                  }
                  frame True {
                    n158 = Wait (ms)(milliseconds to wait=w381) -> ()  [unwired: 1 out]
                  }
                }
              }
            }
            n159 = local read "Move Bias"() -> (w340:dbl)
            n160 = call <userlib>:"BiasSpectroscopy Start.vi"("Application ref in"=w344, "Get data (F)"=TRUE ("Get Data (F)"), "Error in (no error)"=w361) -> ("Application ref out"=w333:refnum<vi>, "Data"=w360:sgl[][], "Parameters"=w359:sgl[], "Error out"=w352:errorcluster)  [unwired: 8 in, 1 out]
            n161 = call <userlib>:"Lockin Mod on_off Set.vi"("Lockin ON/OFF"=FALSE, "Application ref in"=w333) -> ("Application ref out"=w332:refnum<vi>)  [unwired: 8 in, 1 out]
            n162 = call <userlib>:"Voltage Set.vi"("Bias (V)"=w340, "Application ref in"=w332) -> ("Application ref out"=w335:refnum<vi>)  [unwired: 8 in, 1 out]
            n163 = local read "Move Current"() -> (w339:dbl)
            n164 = Delete From Array(array=w360, length=1, index (row)=0 ("index")) -> (array with subset deleted=w358:sgl[][])  [unwired: 1 in, 1 out]
            n165 = call <userlib>:"Ctrl-on_off Set.vi"("Z Controller ON/OFF"=TRUE, "Application ref in"=w335) -> ("Application ref out"=w334:refnum<vi>)  [unwired: 8 in, 1 out]
            n166 = Write to Binary File(file (use dialog)=w364, data=w359, error in=w352, 5:FALSE ("prepend array or string size? (T)")) -> (refnum out=w363:refnum<file>, error out=w351:errorcluster)  [unwired: 2 in, 1 out]
            n167 = call <userlib>:"Z-Ctrl Setpoint Set.vi"("Z Controller setpoint"=w339, "Application ref in"=w334) -> ("Application ref out"=w341:refnum<vi>)  [unwired: 8 in, 1 out]
            n168 = Increment(x=w349) -> (x+1=w348:i32)
            n169 = Write to Binary File(file (use dialog)=w363, data=w358, error in=w351, 5:FALSE ("prepend array or string size? (T)")) -> (refnum out=w362:refnum<file>, error out=w350:errorcluster)  [unwired: 2 in, 1 out]
          }
        }
        n170 = Get Date/Time In Seconds() -> (seconds since 1Jan1904=w179:timestamp)
        n171 = local read "total Points"() -> (w185:i32)
        n172 = Subtract(x=w179, y=w184) -> (x-y=w183:dbl)
        n173 = Divide(x=w182, y=w185) -> (x/y=w188:dbl)
        n174 = Subtract(x=w185, y=w182) -> (x-y=w180:i32)
        n175 = Divide(x=w183, y=w182) -> (x/y=w181:dbl)
        n176 = Multiply(x=w181, y=w180) -> (x*y=w178:dbl)
        "remaining" <- w178
        n177 = Multiply(x=w188, y=100.0) -> (x*y=→"Progress":dbl)
        n178 = Add(x=w179, y=w178) -> (x+y=→"ETA":timestamp)
      }
      frame "end" {
        n179 = Close File(refnum=w412) -> ()  [unwired: 1 in, 2 out]
        n180 = Close File(refnum=w410) -> (path=w409:path)  [unwired: 1 in, 1 out]
        n181 = local write "Status"("finishing" ("Status")) -> ()
        n182 = call "STSGrid.vi"("Binary Spectroscopy File"=w409) -> ()  [unwired: 11 in]
        n183 = Bundle(w417, w417) -> (w439:cluster{sgl[][], sgl[][]})  [unwired: 1 in]
        n184 = Build Array(w439) -> (w438:cluster{sgl[][], sgl[][]}[])
        n185 = Unbundle By Name(w427) -> ("center X (m)"=w425:sgl, "center Y (m)"=w424:sgl, "angle (deg)"=w423:sgl, "width (m)"=w422:sgl, "height (m)"=w421:sgl)
        n186 = Strip Path(path=w397) -> (stripped path=w431:path, name=w430:string)
        n187 = Get Date/Time In Seconds() -> (seconds since 1Jan1904=w393:timestamp)
        n188 = Bundle By Name(cluster=T5 {"up/down"=FALSE, "time/line"=0.0, "start time"=timestamp(0 s since 1904-01-01), "end time"=timestamp(0 s since 1904-01-01)} ("Scan param"), "up/down"=TRUE, "time/line"=sgl nan ("input 7"), "start time"=w435, "end time"=w393) -> (w434:T5)
        n189 = Bundle By Name(cluster=T3 {"center X"=0.0, "center Y"=0.0, "angle"=0.0, "width"=0.0, "height"=0.0, "# pixels"=0, "# lines"=0} ("Scanfield"), "center X"=w425, "center Y"=w424, "angle"=w423, "width"=w422, "height"=w421, "# lines"=w418, "# pixels"=w419) -> (w420:T3)
        n190 = Bundle("stripped path"=w431, "name"=w430) -> (w429:cluster{"stripped path":path, "name":string})  [unwired: 1 in]
        n191 = call <userlib>:"Save sxm File.vi"("Auto file naming? (T)"=FALSE, "Scanfield"=w420, "Scan param"=w434, "error in (no error)"=w428, "Channels data"=w438, "Channels config"=T4 [{"Name"="Z (m)", "Calibration"=1.0, "Offset"=0.0, "Channel index"=0}], "Filename control"=w429) -> ("error out"=w404:errorcluster)  [unwired: 2 in, 2 out]
        n192 = Strip Path(path=w397) -> (stripped path=w408:path)  [unwired: 1 out]
        n193 = Strip Path(path=w408) -> (stripped path=w407:path)  [unwired: 1 out]
        n194 = call <userlib>:"Get Session Path.vi"("error in (no error)"=w404, "Application ref in"=w403) -> ("error out"=w400:errorcluster, "Session path"=w402:path, "Application ref out"=w386:refnum<vi>)  [unwired: 7 in]
        n195 = Path To String(path=w397) -> (string=w396:string)
        n196 = Path To String(path=w407) -> (string=w405:string)
        n197 = call "SXM.vi"("Path"=w402, "Delete"=FALSE, "error in"=w400) -> ("error out"=w399:errorcluster)  [unwired: 7 in]
        n198 = call "ChangeSessionV2.vi"("error in (no error)"=w399, "Session"=w405) -> ("error out"=w398:errorcluster)
        n199 = Format Date/Time String(time format string (%c)=" Finished at %y%m%d - %H%M%S ", seconds (now)=w393) -> (date/time string=w392:string)  [unwired: 1 in]
        n200 = Concatenate Strings(w396, "\r\n", w392) -> (w395:string)
        n201 = Search and Replace String(input string="Email when finished", search string="@") -> (number of replacements=w388:i32)  [unwired: 6 in, 3 out]
        n202 = Greater Than 0?(x=w388) -> (x > 0?=w387:bool)
        n203 = case shown="True" w387 {
          tunnel: w398 -> [_ w446]
          tunnel: w395 -> [_ w444]
          tunnel: "Email when finished" -> [_ w443]
          frame False {
          }
          frame True {
            n204 = call "Send Email"("error in"=w446, "Message"=w444, "Subject"="Grid Finished", "Recipients"=w443) -> ()  [unwired: 7 in, 1 out]
          }
        }
        n205 = call <userlib>:"BiasSpectroscopy SetProperties.vi"("Application ref in"=w386, "Z-Controller hold (no change)"=enum16{"no change", "on", "off"}."on") -> ("Application ref out"=w384:refnum<vi>)  [unwired: 12 in, 1 out]
        n206 = call <userlib>:"TipLift Set.vi"("TipLift (m)"=sgl 0.0, "Application ref in"=w384) -> ("Application ref out"=w383:refnum<vi>)  [unwired: 8 in, 1 out]
      }
    }
    "Error out" <- w42
    "Points taken" <- w10
    "X Offset" <- w9
    "Y Offset" <- w8
  }
